vi "Close.vi"(8 "error in (no error)":errorcluster, 11 "object in":refnum<class "TableLogger_SQLite_Actor.lvclass">) -> (0 "error out":errorcluster, 3 "object out":refnum<class "TableLogger_SQLite_Actor.lvclass">)   [LabVIEW 2014, in "TableLogger_SQLite_Actor.lvlib" / "TableLogger_SQLite_Actor.lvclass"]
uses:
  TableLogger_SQLite_Actor.lvclass
  TableLogger_SQLite_Actor.lvclass/TableLogger_SQLite_Actor.ctl
  <vilib>/drjdpowell/SQLite Library/SQL Connection/Connection.lvclass
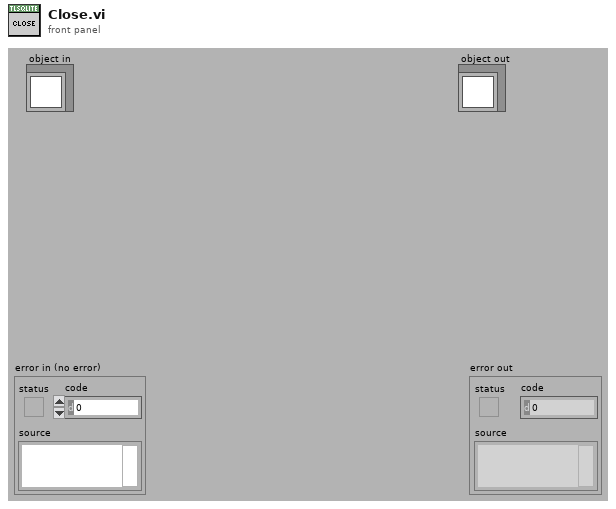
[diagram p1: front panel]
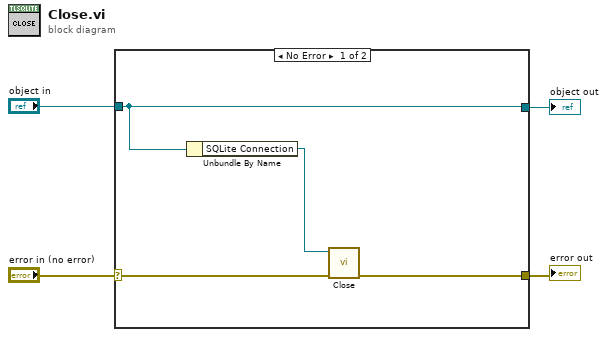
[diagram p0: block diagram]
diagram:
  n1 = case shown="No Error" "error in (no error)" {
    selector: "error in (no error)" -> [w8 w10]
    tunnel: [w6 w10] -> w3
    tunnel: [w7 w9] -> w1
    tunnel: "object in" -> [w7 w9]
    frame No Error {
      n2 = Unbundle By Name(w7) -> ("SQLite Connection"=w5:refnum<class "Connection.lvclass">)
      n3 = call-dynamic "Close.vi"("error in (no error)"=w8, "SQLite Connection in"=w5) -> ("error out"=w6:errorcluster)  [unwired: 9 in]
    }
    frame Error {
    }
  }
  "error out" <- w3
  "object out" <- w1
